vi "kissia_ArduinoMicro Module.vi"(5 "Enable":bool=TRUE, 6 "Timeout(s)":dbl=2.0, 7 "Command":T2, 8 "error in (no error)":errorcluster, 10 "VALVES":T1, 11 "VISA resource name":refnum<visa-resource-name>="COM39") -> (0 "error out":errorcluster, 2 "read string":string, 3 "TimeOut":bool, 4 "write string":string)   [LabVIEW 2017]
uses:
  kissia_ArduinoMicro Module.ctl
  <vilib>/Instr/_visa.llb/VISA Configure Serial Port (Instr).vi
panel:
  out "Bytes at Serial Port":u32
  # "Output Data"
  # "Input Data"
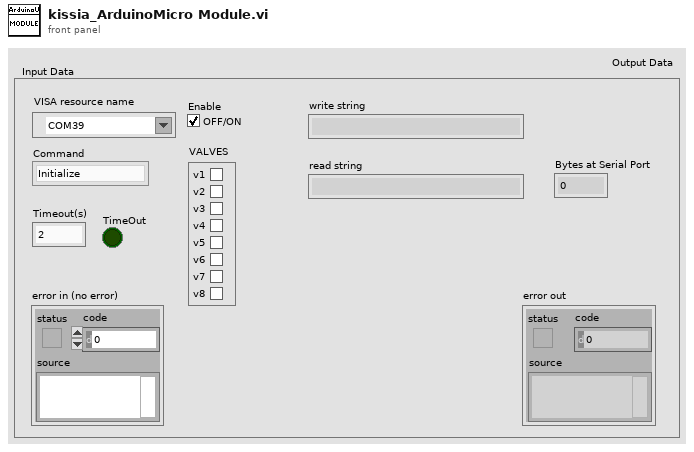
[diagram p1: front panel]
types:
  T1 = cluster{"v1":bool, "v2":bool, "v3":bool, "v4":bool, "v5":bool, "v6":bool, "v7":bool, "v8":bool}
  T2 = typedef "kissia_ArduinoMicro Module.ctl" = enum16{"Initialize", "Read Data", "Write Data", "Enable", "Disable", "Shutdown"}
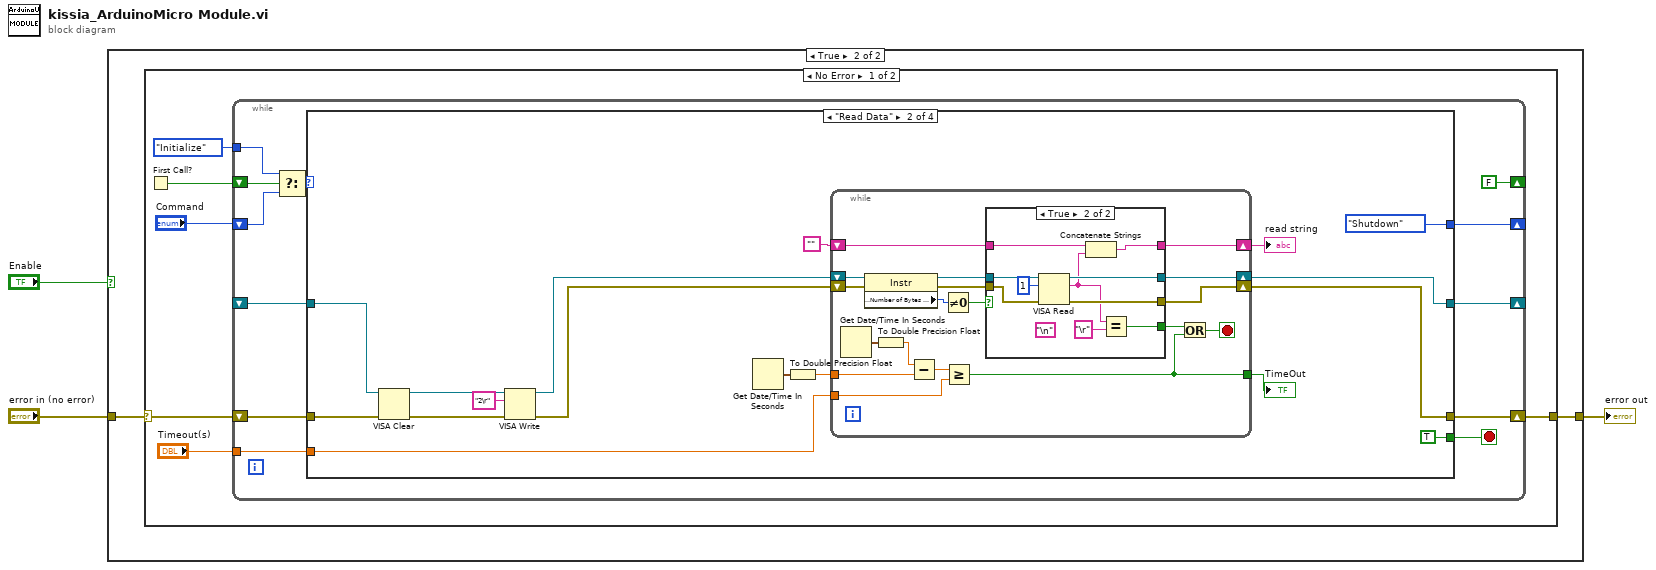
[diagram p0: block diagram]
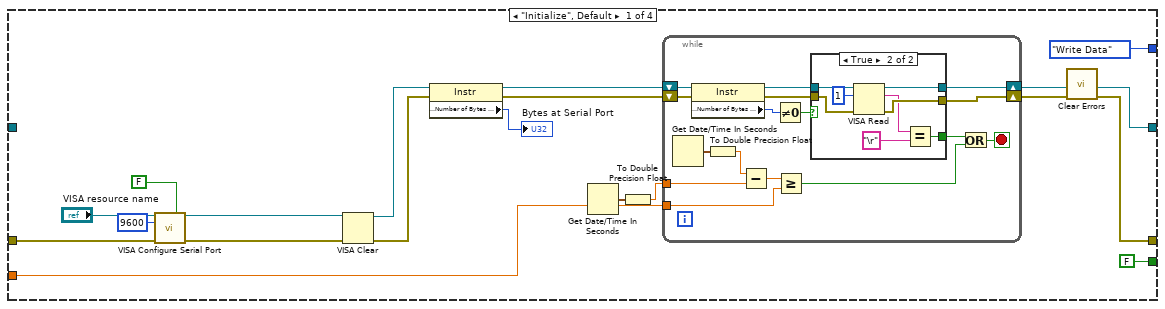
[diagram p3: hidden frame]
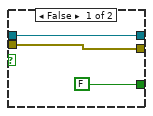
[diagram p4: hidden frame]
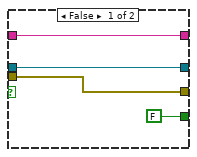
[diagram p5: hidden frame]
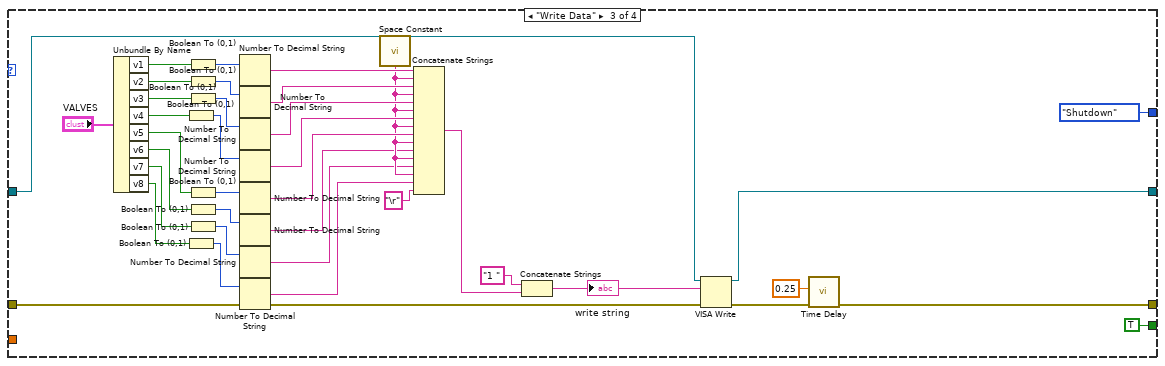
[diagram p6: hidden frame]
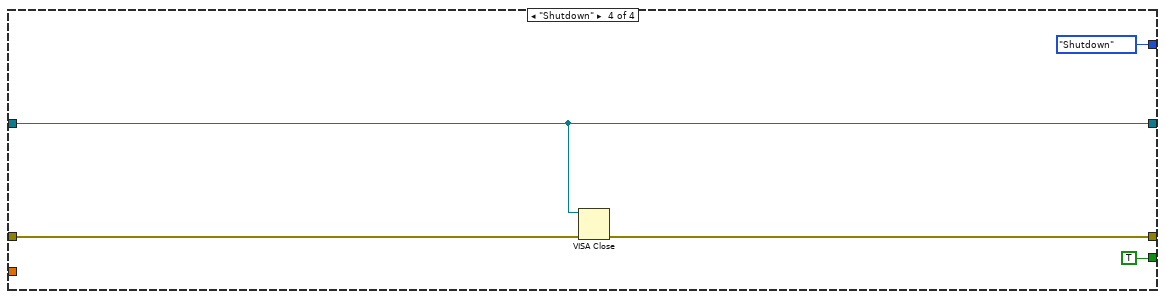
[diagram p7: hidden frame]
diagram:
  n1 = case shown="True" "Enable" {
    tunnel: "error in (no error)" -> [w4 w6]
    tunnel: [w4 w5] -> w2
    frame False {
    }
    frame True {
      n2 = case shown="No Error" w6 {
        selector: w6 -> [w10 w163]
        tunnel: [w9 w163] -> w5
        frame No Error {
          n3 = First Call?() -> (First Call?: T/F=w12:bool)
          n4 = while {
            shift-right: [w15] -> _
            shift-left: "Command" -> [w21]
            shift-right: [w18] -> w9
            shift-left: w10 -> [w19]
            shift-right: [FALSE ("First Call?: T/F")] -> _
            shift-left: w12 -> [w24]
            tunnel: kissia_ArduinoMicro_Module."Initialize" ("t") -> [w23]
            shift-right: [w17] -> _
            shift-left: _ -> [w16]
            tunnel: "Timeout(s)" -> [w13]
            stop <- w14 stop-if-true
            n5 = Select(t=w23, s=w24, f=w21) -> (s? t:f=w20:T2)
            n6 = case shown="\"Read Data\"" w20 {
              tunnel: w19 -> [w38 w78 w157 w159]
              tunnel: [w29 w79 w138 w158] -> w18
              tunnel: [w34 w80 w154 w160] -> w17
              tunnel: w16 -> [_ w77 w130 w160]
              tunnel: [kissia_ArduinoMicro_Module."Write Data" ("t") kissia_ArduinoMicro_Module."Shutdown" ("t") kissia_ArduinoMicro_Module."Shutdown" ("t") kissia_ArduinoMicro_Module."Shutdown" ("t")] -> w15
              tunnel: [FALSE ("Enable Termination\nChar (T)") TRUE ("Enable Termination\nChar (T)") TRUE ("Enable Termination\nChar (T)") TRUE ("Enable Termination\nChar (T)")] -> w14
              tunnel: w13 -> [w33 w83 _ _]
              frame "Initialize", Default {
                n7 = call-poly "VISA Configure Serial Port"("VISA resource name"="VISA resource name", "Enable Termination\nChar (T)"=FALSE ("Enable Termination\nChar (T)"), "baud rate (9600)"=u32 9600, "error in (no error)"=w38) -> ("VISA resource name out"=w32:refnum<visa-resource-name>, "error out"=w31:errorcluster)  [unwired: 10 in]
                n8 = VISA Clear(VISA resource name=w32, error in (no error)=w31) -> (VISA resource name out=w26:refnum<visa-resource-name>, error out=w28:errorcluster)
                n9 = property class="Instr"(reference=w26, error in=w28) -> (reference out=w25:refnum<visa-resource-name>, error out=w27:errorcluster, "Serial Settings:Number of Bytes at Serial Port"=→"Bytes at Serial Port":u32)
                n10 = Get Date/Time In Seconds() -> (seconds since 1Jan1904=w37:timestamp)
                n11 = To Double Precision Float(number=w37) -> (double precision float=w36:dbl)
                n12 = while {
                  tunnel: w36 -> [w44]
                  shift-right: [w54] -> w34
                  shift-left: w25 -> [w52]
                  shift-right: [w53] -> w35
                  shift-left: w27 -> [w51]
                  tunnel: w33 -> [w45]
                  stop <- w59 stop-if-true
                  n13 = Get Date/Time In Seconds() -> (seconds since 1Jan1904=w58:timestamp)
                  n14 = property class="Instr"(reference=w52, error in=w51) -> (reference out=w49:refnum<visa-resource-name>, error out=w50:errorcluster, "Serial Settings:Number of Bytes at Serial Port"=w48:u32)
                  n15 = To Double Precision Float(number=w58) -> (double precision float=w57:dbl)
                  n16 = Subtract(x=w57, y=w44) -> (x-y=w56:dbl)
                  n17 = Not Equal To 0?(x=w48) -> (x != 0?=w47:bool)
                  n18 = Greater Or Equal?(x=w56, y=w45) -> (x >= y?=w55:bool)
                  n19 = case shown="True" w47 {
                    tunnel: [w62 w70] -> w54
                    tunnel: [w61 w69] -> w53
                    tunnel: w50 -> [w61 w68]
                    tunnel: w49 -> [w62 w67]
                    tunnel: [FALSE w64] -> w46
                    frame False {
                    }
                    frame True {
                      n20 = VISA Read(VISA resource name=w67, byte count=u32 1, error in (no error)=w68) -> (VISA resource name out=w70:refnum<visa-resource-name>, read buffer=w65:string, error out=w69:errorcluster)  [unwired: 1 out]
                      n21 = Equal?(x=w65, y="\r" ("Mide")) -> (x = y?=w64:bool)
                    }
                  }
                  n22 = Or(x=w46, y=w55) -> (x .or. y?=w59:bool)
                }
                n23 = call <vilib>:"Clear Errors.vi"("error in (no error)"=w35) -> ("error out"=w29:errorcluster)  [unwired: 5 in, 1 out]
              }
              frame "Read Data" {
                n24 = VISA Clear(VISA resource name=w77, error in (no error)=w78) -> (VISA resource name out=w75:refnum<visa-resource-name>, error out=w73:errorcluster)
                n25 = VISA Write(VISA resource name=w75, write buffer="2\r", error in (no error)=w73) -> (VISA resource name out=w74:refnum<visa-resource-name>, error out=w72:errorcluster)  [unwired: 1 out]
                n26 = Get Date/Time In Seconds() -> (seconds since 1Jan1904=w82:timestamp)
                n27 = To Double Precision Float(number=w82) -> (double precision float=w81:dbl)
                n28 = while {
                  tunnel: w81 -> [w102]
                  shift-right: [w98] -> w80
                  shift-left: w74 -> [w96]
                  shift-right: [w97] -> w79
                  shift-left: w72 -> [w95]
                  tunnel: w83 -> [w100]
                  tunnel: [w99] -> w84
                  shift-right: [w89] -> w76
                  shift-left: "" -> [w90]
                  stop <- w105 stop-if-true
                  n29 = Get Date/Time In Seconds() -> (seconds since 1Jan1904=w104:timestamp)
                  n30 = property class="Instr"(reference=w96, error in=w95) -> (reference out=w93:refnum<visa-resource-name>, error out=w94:errorcluster, "Serial Settings:Number of Bytes at Serial Port"=w92:u32)
                  n31 = To Double Precision Float(number=w104) -> (double precision float=w103:dbl)
                  n32 = Subtract(x=w103, y=w102) -> (x-y=w101:dbl)
                  n33 = Not Equal To 0?(x=w92) -> (x != 0?=w91:bool)
                  n34 = Greater Or Equal?(x=w101, y=w100) -> (x >= y?=w99:bool)
                  n35 = case shown="True" w91 {
                    tunnel: [w109 w119] -> w98
                    tunnel: [w108 w118] -> w97
                    tunnel: w94 -> [w108 w117]
                    tunnel: w93 -> [w109 w116]
                    tunnel: w90 -> [w107 w115]
                    tunnel: [w107 w114] -> w89
                    tunnel: [FALSE w111] -> w88
                    frame False {
                    }
                    frame True {
                      (unwired) "\n"
                      n36 = VISA Read(VISA resource name=w116, byte count=u32 1, error in (no error)=w117) -> (VISA resource name out=w119:refnum<visa-resource-name>, read buffer=w112:string, error out=w118:errorcluster)  [unwired: 1 out]
                      n37 = Concatenate Strings(w115, w112) -> (w114:string)
                      n38 = Equal?(x=w112, y="\r" ("Mide")) -> (x = y?=w111:bool)
                    }
                  }
                  n39 = Or(x=w88, y=w99) -> (x .or. y?=w105:bool)
                }
                "read string" <- w76
                "TimeOut" <- w84
              }
              frame "Write Data" {
                n40 = Unbundle By Name("VALVES") -> ("v1"=w152:bool, "v2"=w151:bool, "v3"=w150:bool, "v4"=w149:bool, "v5"=w129:bool, "v6"=w128:bool, "v7"=w127:bool, "v8"=w126:bool)
                n41 = Boolean To (0,1)(Boolean=w149) -> (0, 1=w144:i16)
                n42 = Boolean To (0,1)(Boolean=w126) -> (0, 1=w134:i16)
                n43 = Boolean To (0,1)(Boolean=w152) -> (0, 1=w148:i16)
                n44 = Boolean To (0,1)(Boolean=w151) -> (0, 1=w146:i16)
                n45 = Boolean To (0,1)(Boolean=w150) -> (0, 1=w145:i16)
                n46 = Boolean To (0,1)(Boolean=w129) -> (0, 1=w131:i16)
                n47 = Boolean To (0,1)(Boolean=w128) -> (0, 1=w132:i16)
                n48 = Boolean To (0,1)(Boolean=w127) -> (0, 1=w133:i16)
                n49 = Number To Decimal String(number=w148) -> (decimal integer string=w147:string)  [unwired: 1 in]
                n50 = Number To Decimal String(number=w146) -> (decimal integer string=w143:string)  [unwired: 1 in]
                n51 = Number To Decimal String(number=w145) -> (decimal integer string=w142:string)  [unwired: 1 in]
                n52 = Number To Decimal String(number=w144) -> (decimal integer string=w141:string)  [unwired: 1 in]
                n53 = Number To Decimal String(number=w131) -> (decimal integer string=w125:string)  [unwired: 1 in]
                n54 = Number To Decimal String(number=w132) -> (decimal integer string=w123:string)  [unwired: 1 in]
                n55 = Number To Decimal String(number=w133) -> (decimal integer string=w122:string)  [unwired: 1 in]
                n56 = Number To Decimal String(number=w134) -> (decimal integer string=w121:string)  [unwired: 1 in]
                n57 = call <vilib>:"Space Constant.vi"() -> ("String"=w124:string)
                n58 = Concatenate Strings(w147, w124, w143, w124, w142, w124, w141, w124, w125, w124, w123, w124, w122, w124, w121, "\r" ("string")) -> (w136:string)
                n59 = Concatenate Strings("1 " ("write buffer"), w136) -> (w135:string)
                "write string" <- w135
                n60 = VISA Write(VISA resource name=w130, write buffer=w135, error in (no error)=w157) -> (VISA resource name out=w154:refnum<visa-resource-name>, error out=w139:errorcluster)  [unwired: 1 out]
                n61 = call "Time Delay"("error in (no error)"=w139, "Delay Time (s)"=0.25) -> ("error out"=w138:errorcluster)  [unwired: 9 in]
              }
              frame "Shutdown" {
                n62 = VISA Close(VISA resource name=w160, error in (no error)=w159) -> (error out=w158:errorcluster)
              }
            }
          }
        }
        frame Error {
        }
      }
    }
  }
  "error out" <- w2
